vi "多参数全局变量.vi"() -> ()   [LabVIEW 2016, in "斯坦道多参数.lvlib"]
uses:
  <vilib>/Plasmionique/MB Master/MB_Master_Serial/MB_Master_Serial.lvclass
panel:
  in  "运行模式":enum16{"维护模式", "常规模式", "应急模式", "质控模式"}(ring)=enum."常规模式"
  in  "多参数编号":string
  out "藻密度显示":cluster{"温度测量值":sgl, "测量值":sgl, "温度偏移修正值":sgl}
  out "蓝绿藻显示":cluster{"温度测量值":sgl, "测量值":sgl, "温度偏移修正值":sgl}
  out "cond显示":cluster{"温度测量值":sgl, "测量值":sgl, "温度偏移修正值":sgl}
  out "盐度显示":cluster{"温度测量值":sgl, "测量值":sgl, "温度偏移修正值":sgl}
  out "spcond显示":cluster{"温度测量值":sgl, "测量值":sgl, "温度偏移修正值":sgl}
  out "ph显示":cluster{"温度测量值":sgl, "测量值":sgl, "温度偏移修正值":sgl}
  out "水温显示":cluster{"CH":u16, "监测值":dbl, "温度偏移修正值":sgl}={"CH"=1, "监测值"=0.0, "温度偏移修正值"=0.0} {"CH" items=["NULL", "pH", "Cond", "DO", "Turb"]}
  out "浊度显示":cluster{"温度测量值":sgl, "测量值":sgl, "温度偏移修正值":sgl}
  out "DO显示":T1
  out "叶绿素a显示":cluster{"温度测量值":sgl, "测量值":sgl, "温度偏移修正值":sgl}
  out "多参数运行状态":u16(ring) items=["空闲", "水样测试", "标样核查"]
  in  "MB_Serial session":refnum<class "MB_Master_Serial.lvclass">
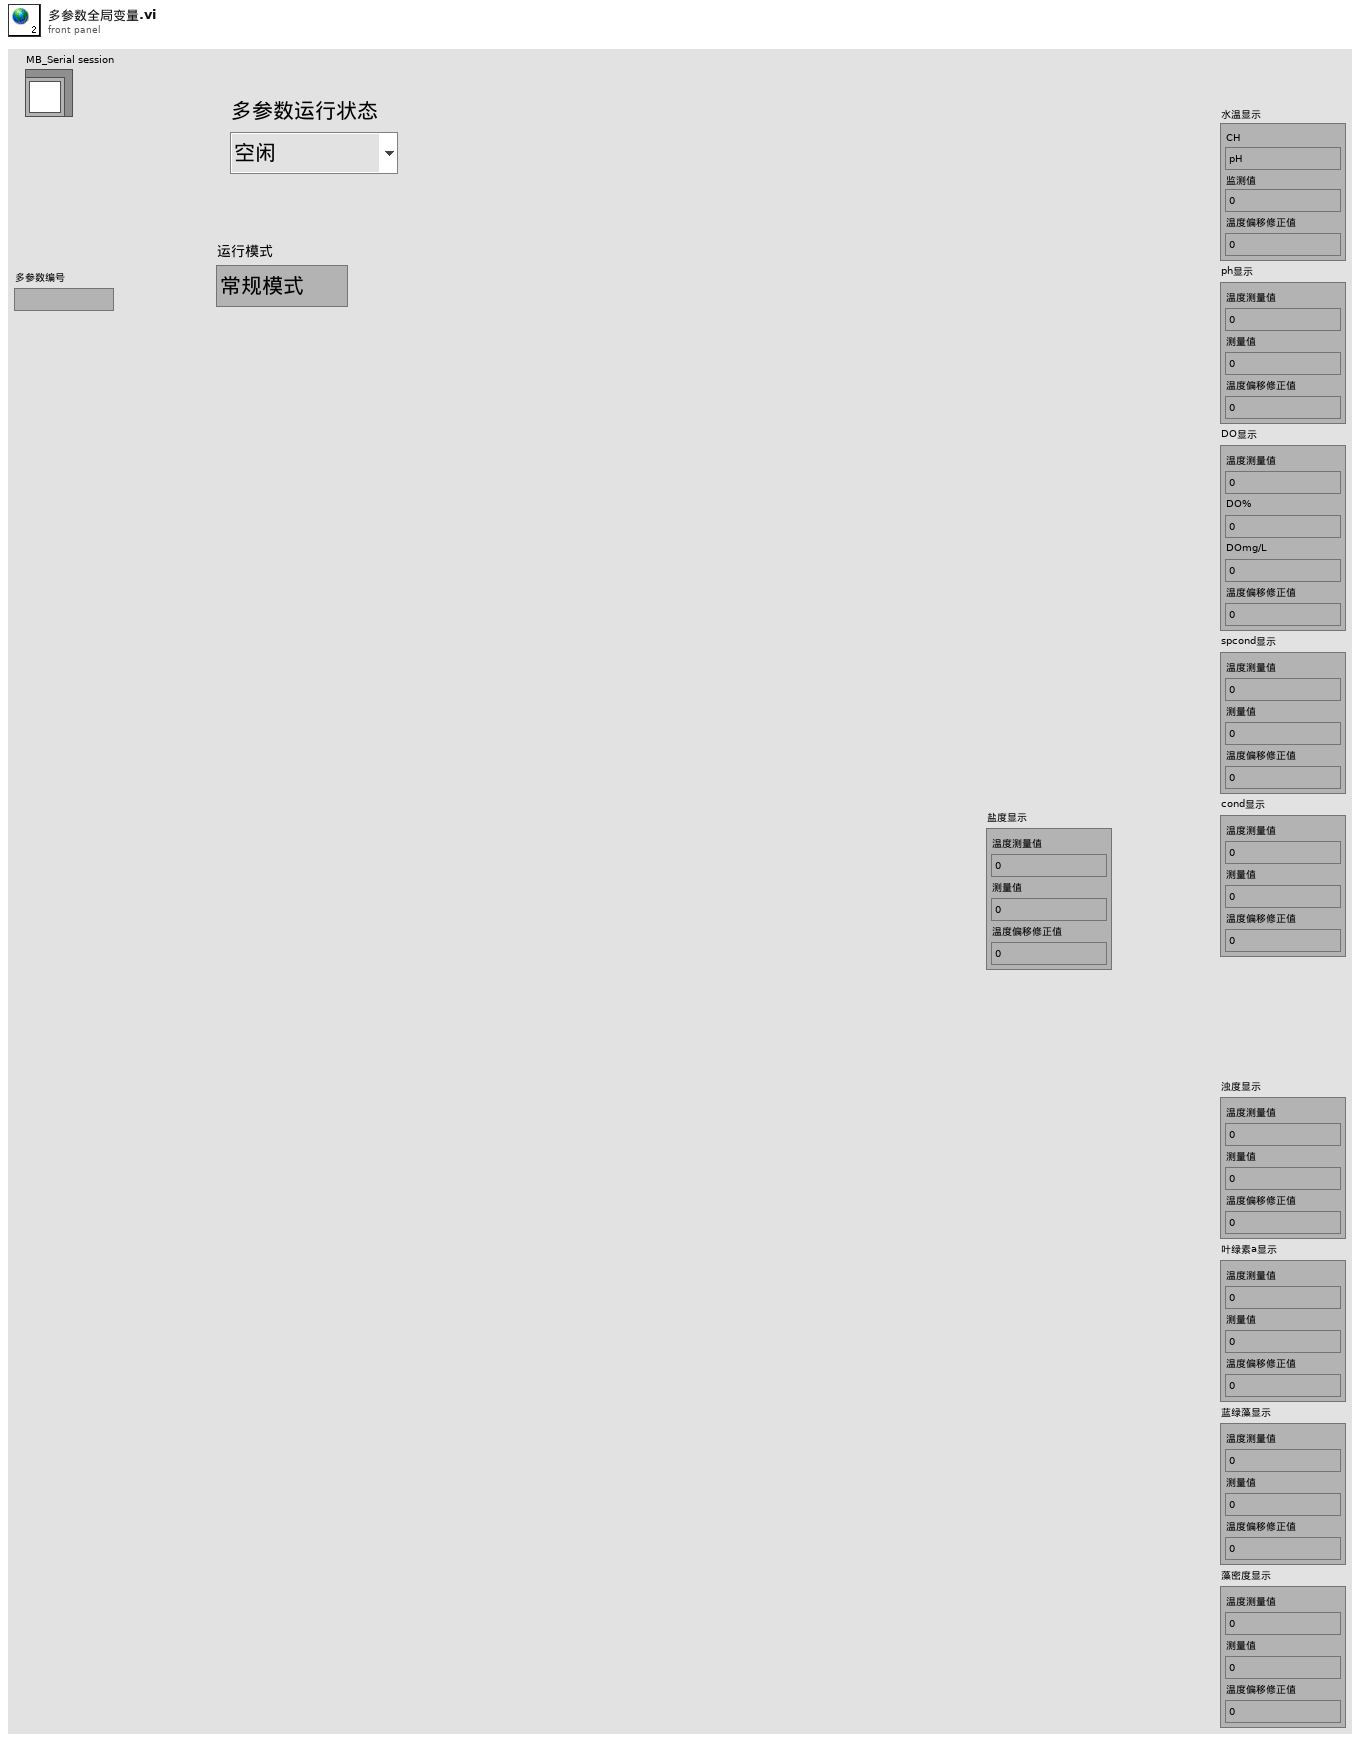
[diagram p1: front panel]
types:
  T1 = cluster{"温度测量值":sgl, "DO%":sgl, "DOmg/L":sgl, "温度偏移修正值":sgl}
diagram:
